vi "2-input OR.vi"(10 "Obtained Expression":string, 11 "Input List":string[](array[string])) -> (1 "O/p = I/p":string, 2 "OR ?":bool, 3 "Logic Exp":string)   [LabVIEW 2014]
doc: "This VI is used to compare the obtained logic with the logic of NAND gate."
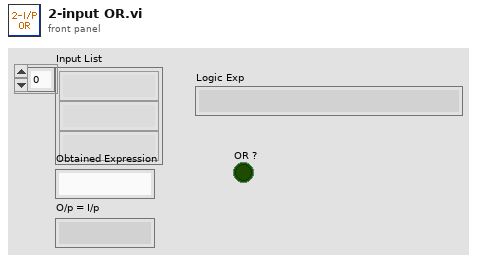
[diagram p1: front panel]
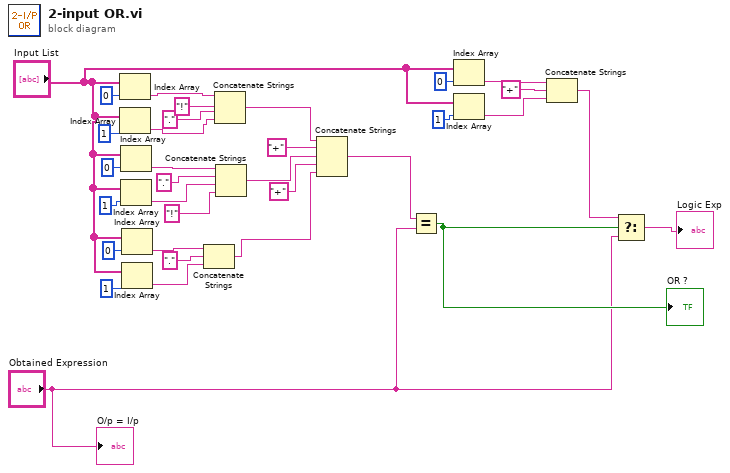
[diagram p0: block diagram]
diagram:
  n1 = Index Array(array="Input List", index=0) -> (element=w17:string)
  n2 = Index Array(array="Input List", index=1) -> (element=w19:string)
  n3 = Index Array(array="Input List", index=0) -> (element=w24:string)
  n4 = Index Array(array="Input List", index=1) -> (element=w22:string)
  n5 = Index Array(array="Input List", index=0) -> (element=w30:string)
  n6 = Index Array(array="Input List", index=1) -> (element=w32:string)
  n7 = Concatenate Strings(w30, "." ("string"), w32) -> (w33:string)
  n8 = Concatenate Strings(w17, "!" ("t"), "." ("string"), w19) -> (w20:string)
  n9 = Concatenate Strings(w24, "." ("string"), w22, "!" ("t")) -> (w26:string)
  n10 = Concatenate Strings(w20, "+" ("string"), w26, "+" ("string"), w33) -> (w14:string)
  n11 = Equal?(x=w14, y="Obtained Expression") -> (x = y?=w13:bool)
  "OR ?" <- w13
  n12 = Index Array(array="Input List", index=0) -> (element=w9:string)
  n13 = Index Array(array="Input List", index=1) -> (element=w7:string)
  n14 = Concatenate Strings(w9, "+" ("string"), w7) -> (w6:string)
  n15 = Select(t=w6, s=w13, f="Obtained Expression") -> (s? t:f=→"Logic Exp":string)
  "O/p = I/p" <- "Obtained Expression"
